vi "get_ini_nxsp.vi"(8 "juese":string, 9 "yw":string, 10 "id":string, 11 "zc_luodi_num":string) -> (3 "sp_gonghao":string)   [LabVIEW 2017, in "Lib_code.lvlib"]
uses:
  Lib_code.lvlib
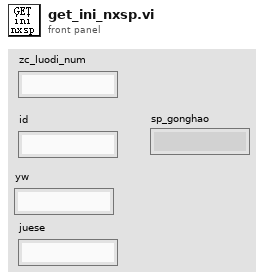
[diagram p1: front panel]
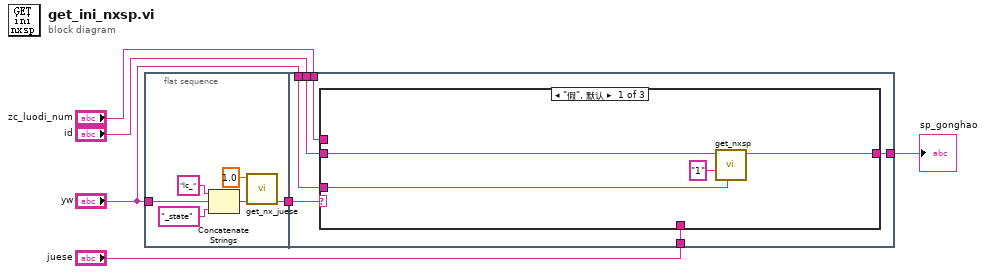
[diagram p0: block diagram]
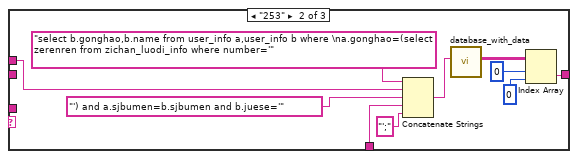
[diagram p2: hidden frame]
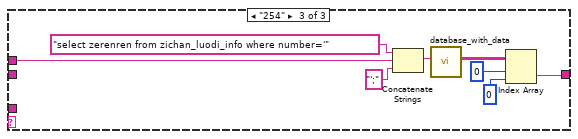
[diagram p3: hidden frame]
diagram:
  n1 = flat-sequence {
    tunnel: "yw" -> [w8]
    tunnel: [w7] -> w5
    tunnel: [w14] -> w6
    tunnel: w5 -> [w18]
    tunnel: "zc_luodi_num" -> [w17]
    tunnel: "id" -> [w16]
    tunnel: "yw" -> [w15]
    tunnel: "juese" -> [w13]
    frame #0 {
      n2 = Concatenate Strings("lc_" ("字符串"), w8, "_state" ("字符串")) -> (w10:string)
      n3 = call "get_nx_juese.vi"("data_name"=w10, "state"=1.0) -> ("nx_juese"=w7:string)  [unwired: 8 in, 1 out]
    }
    frame #1 {
      n4 = case shown="\"假\", 默认" w18 {
        tunnel: w17 -> [_ w24 w40]
        tunnel: w16 -> [w21 _ _]
        tunnel: w15 -> [w20 _ _]
        tunnel: [w19 w30 w34] -> w14
        tunnel: w13 -> [_ w26 _]
        frame "假", Default {
          n5 = call "get_nxsp.vi"("yw"=w20, "Cur_state"="1", "fqren"=w21) -> ("sp_gonghao"=w19:string)  [unwired: 6 in, 2 out]
        }
        frame "253" {
          n6 = Concatenate Strings("select b.gonghao,b.name from user_info a,user_info b where \na.gonghao=(select zerenren from zichan_luodi_info where number='" ("Command Text"), w24, "') and a.sjbumen=b.sjbumen and b.juese='" ("字符串"), w26, "';" ("字符串")) -> (w23:string)
          n7 = call "database_with_data.vi"("input"=w23) -> ("Data"=w29:string[][])  [unwired: 9 in, 1 out]
          n8 = Index Array(array=w29, index (row)=0 ("索引 (行)"), index (col)=0 ("禁用的索引 (列)")) -> (element=w30:string)
        }
        frame "254" {
          n9 = Concatenate Strings("select zerenren from zichan_luodi_info where number='" ("字符串"), w40, "';" ("字符串")) -> (w37:string)
          n10 = call "database_with_data.vi"("input"=w37) -> ("Data"=w33:string[][])  [unwired: 9 in, 1 out]
          n11 = Index Array(array=w33, index (row)=0 ("索引 (行)"), index (col)=0 ("禁用的索引 (列)")) -> (element=w34:string)
        }
      }
    }
  }
  "sp_gonghao" <- w6
